vi "Logging Enabled Page.vi"(8 "error in (no error)":errorcluster, 11 "Node Ptr":T1 format="%.0x") -> (0 "error out":errorcluster)   [LabVIEW 2015, in "Waveform Data Logger System Explorer.lvlib"]
uses:
  Waveform Data Logger System Explorer.lvlib
  <vilib>/NI Veristand/Custom Device API/Custom Device Item Ref.ctl
  <vilib>/NI VeriStand/Custom Device API/Custom Device API.lvlib
panel:
  in  "Header 2":cluster{"Section Name":string}={"Section Name"="Channel Settings"}
  in  "Initial Value":bool
  in  "Header":cluster{"Section Name":string}={"Section Name"="Channel Specification"}
  out "Description":string
  out "Name":string
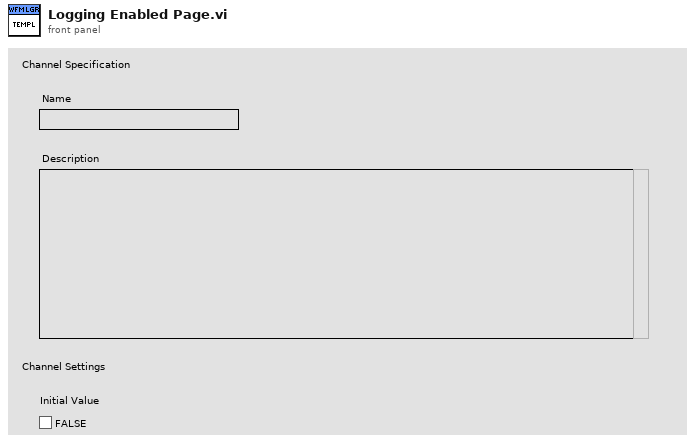
[diagram p1: front panel]
types:
  T1 = typedef "Custom Device API.lvlib/Custom Device Item Ref.ctl" = u64
  T2 = typedef "Custom Device API.lvlib/Custom Device Item Info.ctl" = cluster{"Name":string, "Is Channel":bool, "GUID":string, "Is Waveform":bool}
  T3 = typedef "Custom Device API.lvlib/Custom Device Channel.ctl" = cluster{"Type":T4, "Units":string, "Default Value":dbl, "Faultable":bool, "Scalable":bool}
  T4 = typedef "Custom Device API.lvlib/Custom Device Channel Type.ctl" = enum16{"Input", "Output"}
  T5 = typedef "Custom Device API.lvlib/Custom Device Commands.ctl" = enum16{"Default", "Item renamed", "Shutdown", "Dynamic button pressed"}
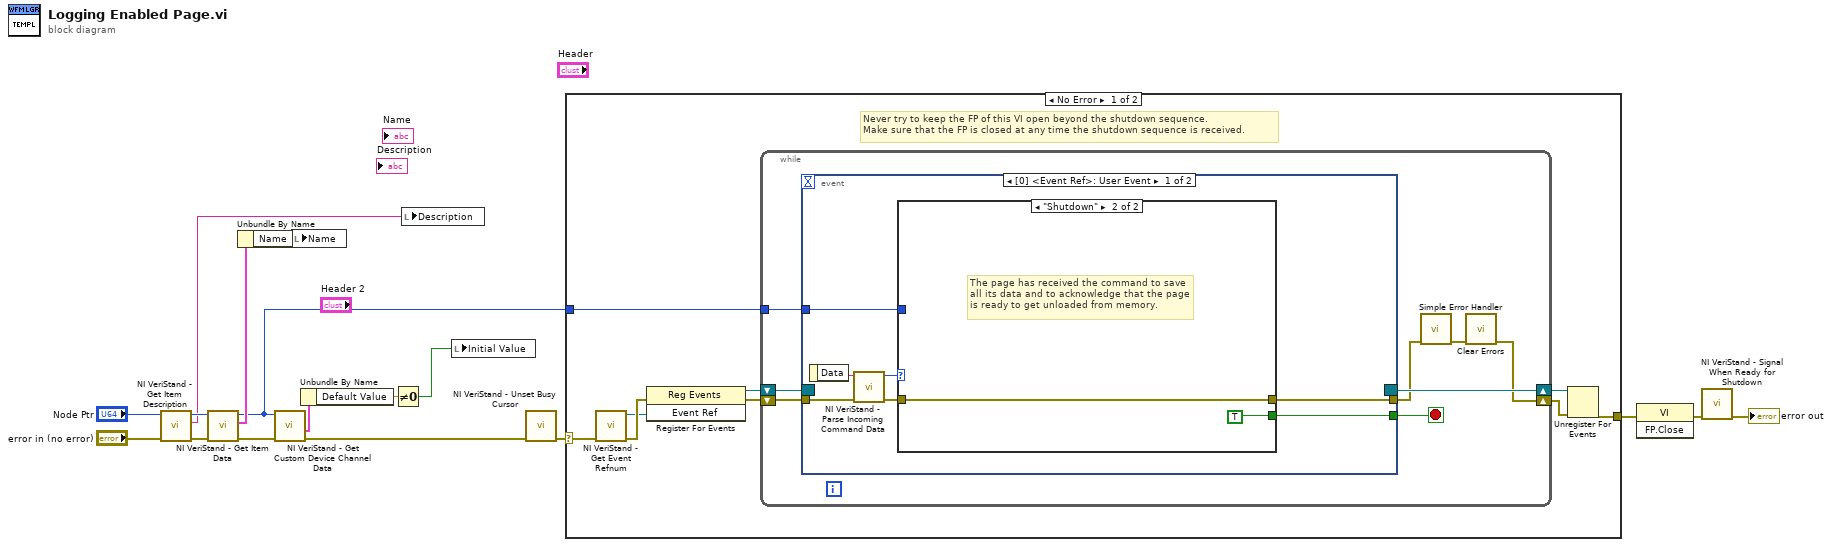
[diagram p0: block diagram]
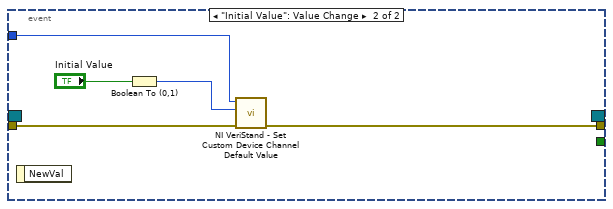
[diagram p3: hidden frame]
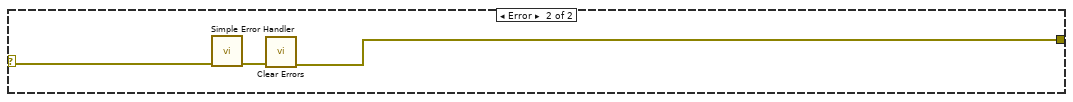
[diagram p4: hidden frame]
diagram:
  n1 = call <vilib>:"NI VeriStand - Get Item Description.vi"("error in (no error)"="error in (no error)", "Item Ref in"="Node Ptr") -> ("error out"=w9:errorcluster, "Description"=w10:string, "Item Ref out"=w11:T1)  [unwired: 7 out]
  n2 = call <vilib>:"NI VeriStand - Get Item Data.vi"("error in (no error)"=w9, "Item Ref in"=w11) -> ("error out"=w6:errorcluster, "Item Info"=w8:T2, "Item Ref out"=w5:T1)  [unwired: 7 out]
  n3 = Unbundle By Name(w8) -> ("Name"=w7:string)
  n4 = call <vilib>:"NI VeriStand - Get Custom Device Channel Data.vi"("error in (no error)"=w6, "Channel Ref in"=w5) -> ("error out"=w4:errorcluster, "Channel"=w3:T3)  [unwired: 8 out]
  n5 = local write "Name"(w7) -> ()
  n6 = Unbundle By Name(w3) -> ("Default Value"=w2:dbl)
  n7 = Not Equal To 0?(x=w2) -> (x != 0?=w1:bool)
  n8 = local write "Description"(w10) -> ()
  n9 = local write "Initial Value"(w1) -> ()
  n10 = call <vilib>:"NI VeriStand - Unset Busy Cursor.vi"("error in (no error)"=w4) -> ("error out"=w13:errorcluster)  [unwired: 10 out]
  n11 = case shown="No Error" w13 {
    selector: w13 -> [w18 w52]
    tunnel: [w23 w50] -> w17
    tunnel: w5 -> [w19 _]
    frame No Error {
      # "Never try to keep the FP of this VI open beyond the shutdown sequence.\nMake sure that the FP is closed at any time the shutdown sequence is received."
      n12 = call <vilib>:"NI VeriStand - Get Event Refnum.vi"("error in (no error)"=w18) -> ("error out"=w26:errorcluster, "Event Ref"=w22:refnum<user-event>)  [unwired: 9 out]
      n13 = register-events(error in=w26, w22) -> (reference out=w20:refnum<event-registration>, error out=w21:errorcluster)  [unwired: 1 in]
      n14 = while {
        tunnel: w19 -> [w30]
        shift-right: [w27] -> w24
        shift-left: w21 -> [w33]
        shift-right: [w34] -> w25
        shift-left: w20 -> [w32]
        stop <- w31 stop-if-true
        n15 = event shown="[0] <Event Ref>: User Event" {
          selector: w32 -> [_ _]
          dyn-events: [_ _] -> w34
          timeout: _ -> [_ _]
          tunnel: w33 -> [w41 w49]
          tunnel: [w37 _] -> w31
          tunnel: [w36 w45] -> w29
          tunnel: w30 -> [w35 w46]
          event User Event {
            n16 = event-data() -> ("Data"=w40:string)  [unwired: 1 out]
            n17 = call <vilib>:"NI VeriStand - Parse Incoming Command Data.vi"("error in (no error)"=w41, "Incoming data"=w40) -> ("error out"=w39:errorcluster, "Action"=w38:T5)  [unwired: 8 out]
            n18 = case shown="\"Shutdown\"" w38 {
              tunnel: w39 -> [w42 w43]
              tunnel: [_ TRUE] -> w37
              tunnel: [w42 w43] -> w36
              tunnel: w35 -> [_ _]
              frame "Default", Default {
              }
              frame "Shutdown" {
                # "The page has received the command to save all its data and to acknowledge that the page is ready to get unloaded from memory."
              }
            }
          }
          event "Initial Value": Value Change {
            n19 = event-data() -> ()  [unwired: 2 out]
            n20 = Boolean To (0,1)(Boolean="Initial Value") -> (0, 1=w47:i16)
            n21 = call <vilib>:"NI VeriStand - Set Custom Device Channel Default Value.vi"("error in (no error)"=w49, "Default Value"=w47, "Channel Ref in"=w46) -> ("error out"=w45:errorcluster)  [unwired: 8 out]
          }
        }
        n22 = call <vilib>:"Simple Error Handler.vi"("error in (no error)"=w29) -> ("error out"=w28:errorcluster)  [unwired: 1 in, 7 out]
        n23 = call <vilib>:"Clear Errors.vi"("error in (no error)"=w28) -> ("error out"=w27:errorcluster)  [unwired: 1 in, 5 out]
      }
      n24 = Unregister For Events(event registration refnum=w25, error in=w24) -> (error out=w23:errorcluster)
    }
    frame Error {
      n25 = call <vilib>:"Simple Error Handler.vi"("error in (no error)"=w52) -> ("error out"=w51:errorcluster)  [unwired: 1 in, 7 out]
      n26 = call <vilib>:"Clear Errors.vi"("error in (no error)"=w51) -> ("error out"=w50:errorcluster)  [unwired: 1 in, 5 out]
    }
  }
  n27 = invoke class="VI" method="FP.Close"(error in=w17) -> (error out=w16:errorcluster)  [unwired: 2 in, 2 out]
  n28 = call <vilib>:"NI VeriStand - Signal When Ready for Shutdown.vi"("error in (no error)"=w16) -> ("error out"=→"error out":errorcluster)  [unwired: 10 out]
